vi "OC_SC_Detection.vi"() -> (2 "Open Loop Channels Array":bool[](array[boolean]), 3 "Short Circuit Channels Array":bool[](array[boolean]))   [LabVIEW 2017, in "BOP_VibAPI_8.lvlib"]
uses:
  <vilib>/addons/InsightCM/Devices/Shared/Cms/Fpga/Acquisition/source/subVIs/VibAPI_8/BOP_VibAPI_8.lvlib
  <vilib>/rvi/eio/common/nirviEmuTemplateMethod_errors.vi
  <vilib>/eio/EIOMethodNode/EIOMethodNode.xnode
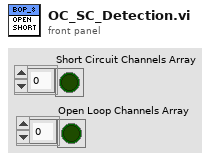
[diagram p1: front panel]
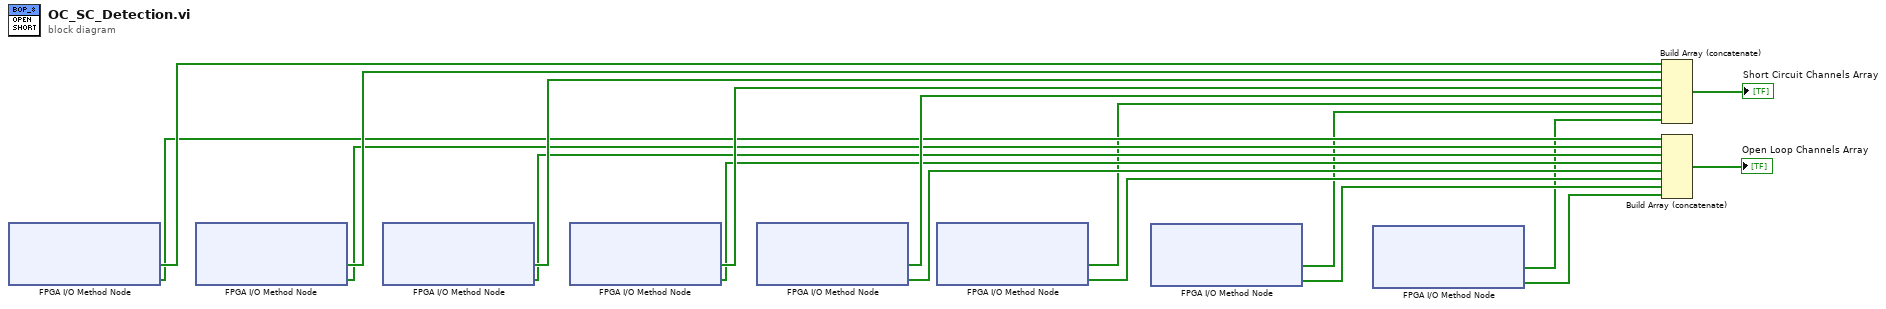
[diagram p0: block diagram]
diagram:
  n1 = xnode "FPGA I/O Method Node"() -> ("Short Circuit"=w18:bool[], "Open Loop"=w13:bool[])  [unwired: 1 in, 1 out]
  n2 = xnode "FPGA I/O Method Node"() -> ("Short Circuit"=w17:bool[], "Open Loop"=w12:bool[])  [unwired: 1 in, 1 out]
  n3 = xnode "FPGA I/O Method Node"() -> ("Short Circuit"=w16:bool[], "Open Loop"=w11:bool[])  [unwired: 1 in, 1 out]
  n4 = xnode "FPGA I/O Method Node"() -> ("Short Circuit"=w15:bool[], "Open Loop"=w10:bool[])  [unwired: 1 in, 1 out]
  n5 = xnode "FPGA I/O Method Node"() -> ("Short Circuit"=w14:bool[], "Open Loop"=w9:bool[])  [unwired: 1 in, 1 out]
  n6 = xnode "FPGA I/O Method Node"() -> ("Short Circuit"=w8:bool[], "Open Loop"=w7:bool[])  [unwired: 1 in, 1 out]
  n7 = xnode "FPGA I/O Method Node"() -> ("Short Circuit"=w4:bool[], "Open Loop"=w3:bool[])  [unwired: 1 in, 1 out]
  n8 = xnode "FPGA I/O Method Node"() -> ("Short Circuit"=w2:bool[], "Open Loop"=w1:bool[])  [unwired: 1 in, 1 out]
  n9 = Build Array (concatenate)(w18, w17, w16, w15, w14, w8, w4, w2) -> (→"Short Circuit Channels Array":bool[])
  n10 = Build Array (concatenate)(w13, w12, w11, w10, w9, w7, w3, w1) -> (→"Open Loop Channels Array":bool[])
